vi "DBVI.vi"(8 "error in (no error)":errorcluster, 10 "ControlQueue":refnum<queue>, 11 "DB in":refnum<class "DB.lvclass">) -> (0 "error out":errorcluster)   [LabVIEW 2015, in "DB.lvclass"]
uses:
  DB.lvclass
  controls/Add.ctl
  controls/Del.ctl
  controls/Update.ctl
  controls/Fix.ctl
  dependecies/ControlsVIs/Clusters-def/Message types.ctl
  Def_DB_FP_ref_commands.ctl
  Def_fix_sql_param.ctl
  GeneralFunctionality/GeneralFunctionality.lvclass/GeneralFunctionality.ctl
  DB.lvclass/DB.ctl
  Message/Message.lvclass/Message.ctl
  dependecies/ControlsVIs/Clusters-def/Standard Command.ctl
  GeneralFunctionality/GeneralFunctionality.lvclass
  Message/Message.lvclass
panel:
  in  "Fix Exp Date":T1
  out "Result Set":string[][](table) caption="Result Set (from first statement with results)"
  in  "SQL command":string
  in  "Fix Users":T1
  in  "Fix Samples":T1=TRUE
  in  "Fix Project":T1=TRUE
  in  "Project Users":string
  in  "Project Date":string caption="Date"
  in  "Project Description":string caption="Description"
  in  "Projects":i16(ring) items=["GNP", "ND"]
  in  "Update project":T2
  in  "Del project":T3
  in  "Add Project":T4
  in  "Project Name":string caption="Name"
  in  "User Date":string caption="Date"
  in  "User  Description":string caption="Description"
  in  "Users":i16(ring) items=["Sergey", "Slava", "Mehran", "Raluca", "Pierre", "Jean-Philippe", "Audrey", "Furong", "Jean-Louis", "Isabelle", "Kash"]
  in  "Update User":T2
  in  "Del User":T3
  in  "Add User":T4
  in  "User name":string caption="Name"
  in  "Exp Date":string caption="Date"
  in  "Exp  Description":string caption="Description"
  in  "Experiments":i16(ring) items=["1-GNP-1_1mM"]
  in  "Update Exp":T2
  in  "Del Exp":T3
  in  "Add Exp":T4
  in  "Exp name":string caption="Name"
  in  "Sample Date":string caption="Date"
  in  "Sample Description":string caption="Description"
  in  "Samples":i16(ring) items=["GNP", "GNP-2mM"]
  in  "Update Sample":T2
  in  "Del Sample":T3
  in  "Add Sample":T4
  in  "Sample Name":string caption="Name"
  out "Received command":string
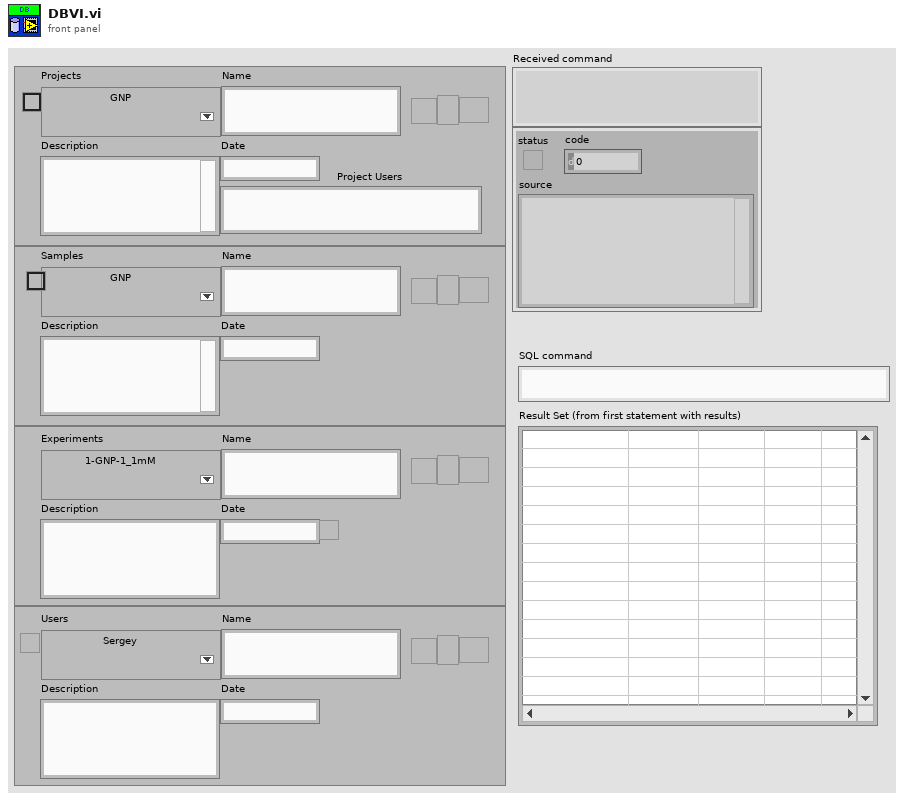
[diagram p1: front panel]
types:
  T1 = typedef "Fix.ctl" = bool
  T2 = typedef "Update.ctl" = bool
  T3 = typedef "Del.ctl" = bool
  T4 = typedef "Add.ctl" = bool
  T5 = typedef "DB.lvclass/Def_fix_sql_param.ctl" = cluster{"Fix Project":bool, "Fix Sample":bool, "Fix Exp Date":bool, "Fix User":bool}
  T6 = typedef "DB.lvclass/Def_DB_FP_ref_commands.ctl" = cluster{"Project Name":refnum<vi>, "Projects":refnum<vi>, "Project Description":refnum<vi>, "Project Date":refnum<vi>, "Project Users":refnum<vi>, "Samples":refnum<vi>, "Sample Name":refnum<vi>, "Sample Description":refnum<vi>, "Sample Date":refnum<vi>, "Experiments":refnum<vi>, "Exp Name":refnum<vi>, "Exp Description":refnum<vi>, "Exp Date":refnum<vi>, "Users":refnum<vi>, "User Name":refnum<vi>, "User Description":refnum<vi>, "User Date":refnum<vi>}
  T7 = typedef "Message types.ctl" = string
  T8 = typedef "Standard Command.ctl" = cluster{"command":string, "data":variant}
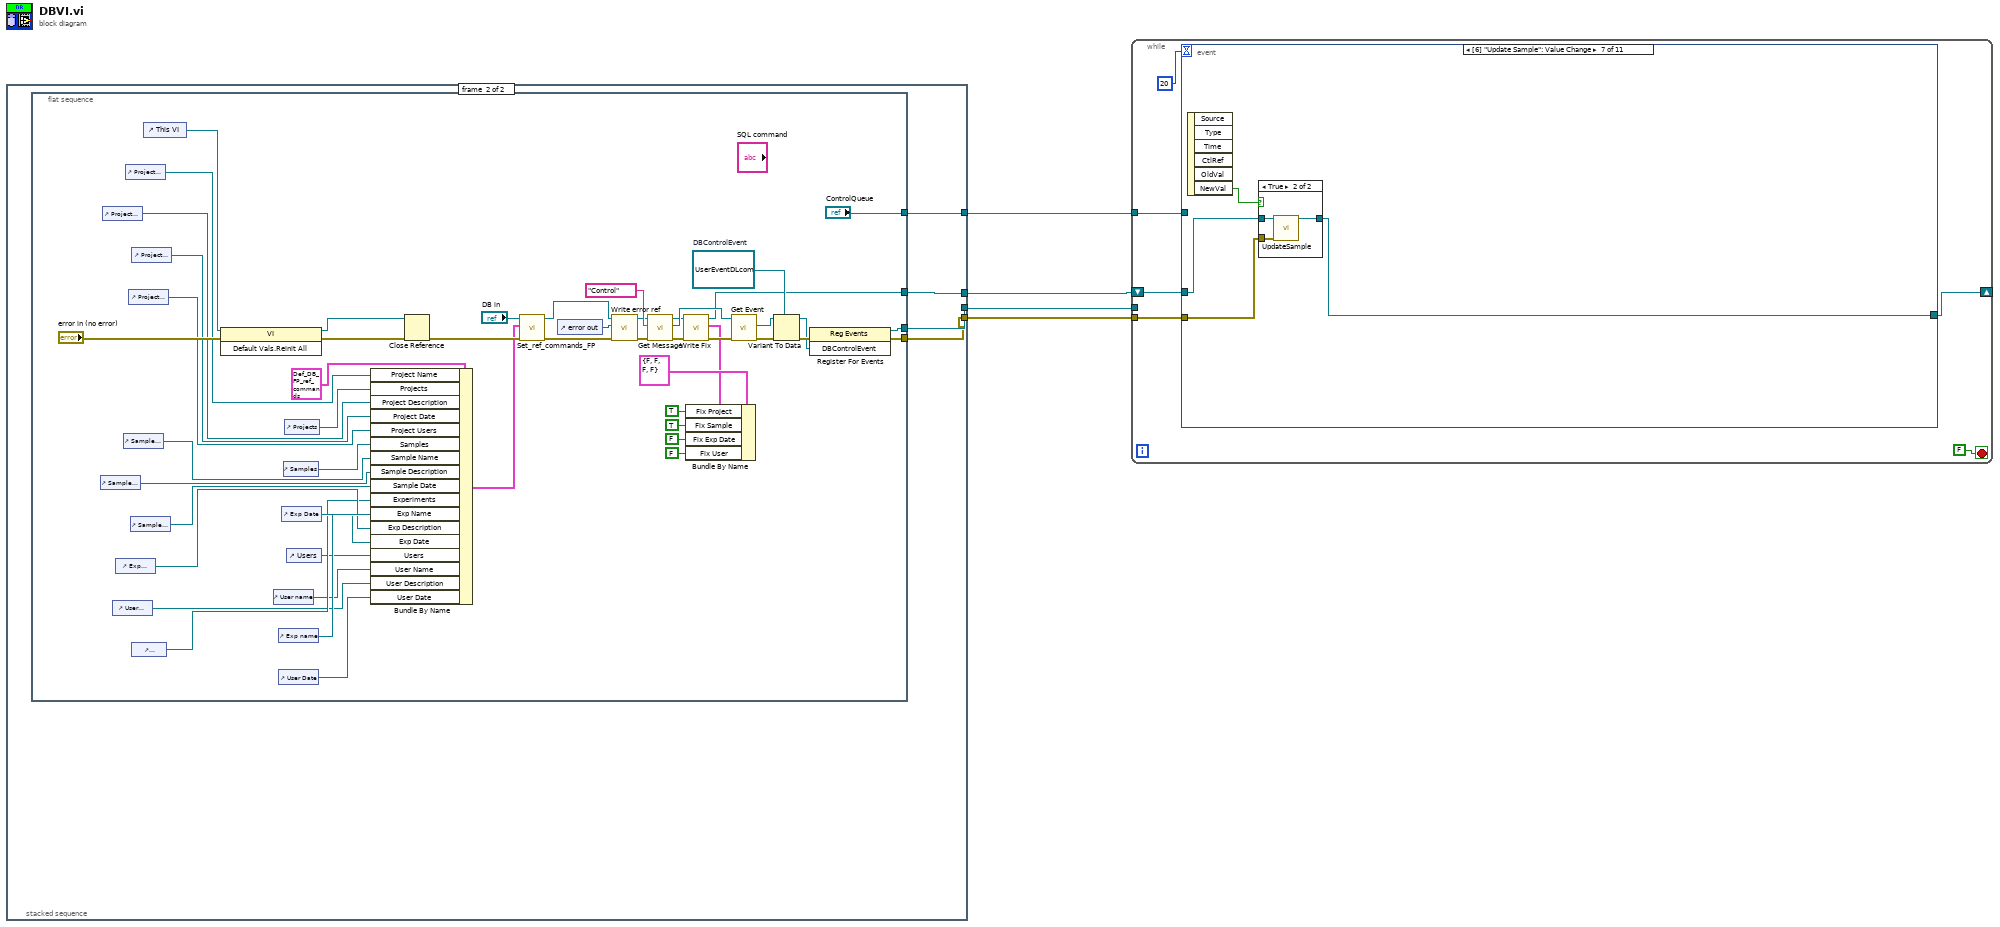
[diagram p0: block diagram]
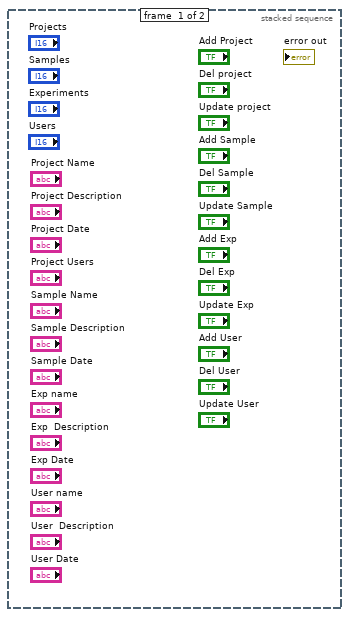
[diagram p2: hidden frame]
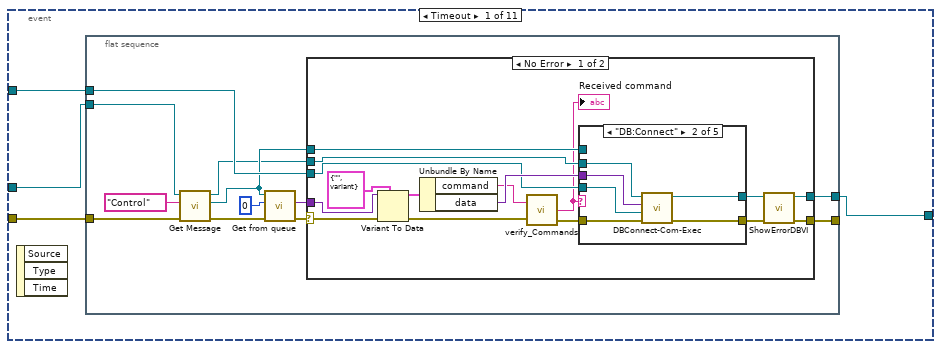
[diagram p3: hidden frame]
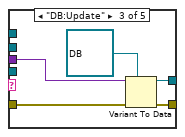
[diagram p5: hidden frame]
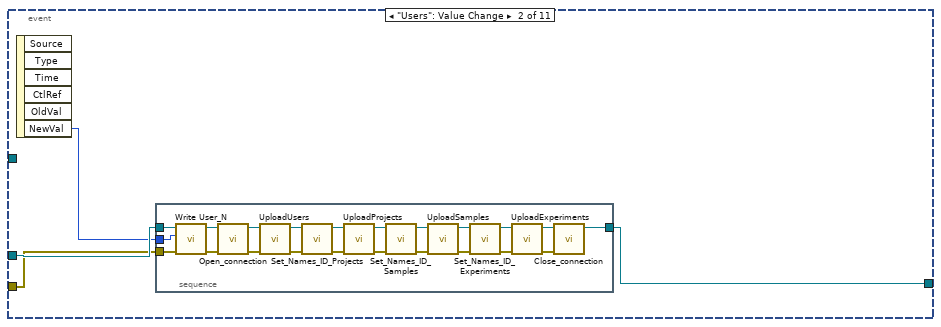
[diagram p9: hidden frame]
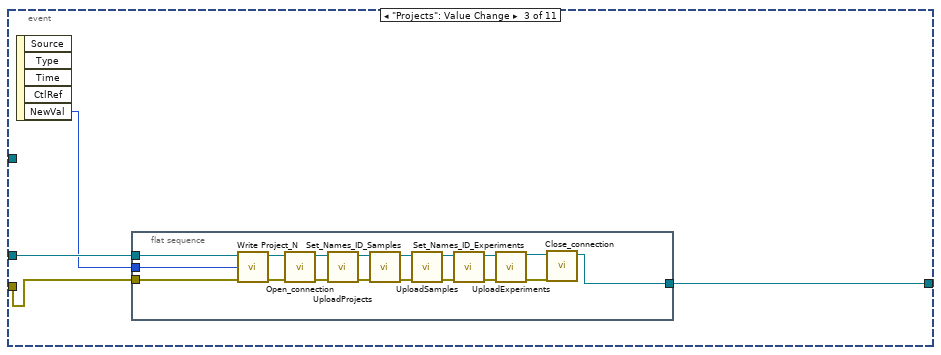
[diagram p10: hidden frame]
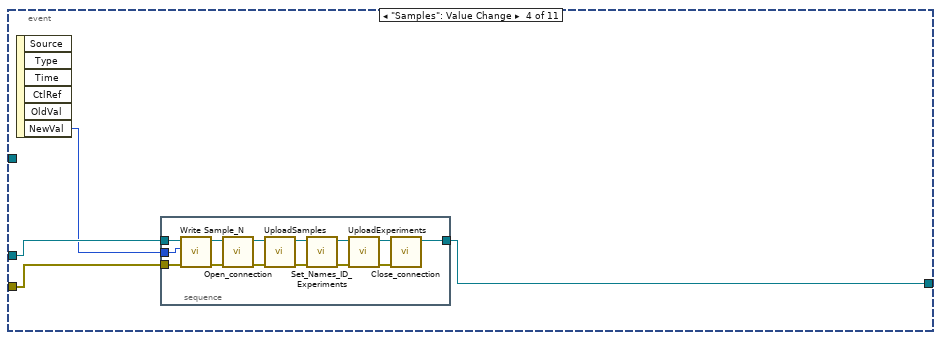
[diagram p11: hidden frame]
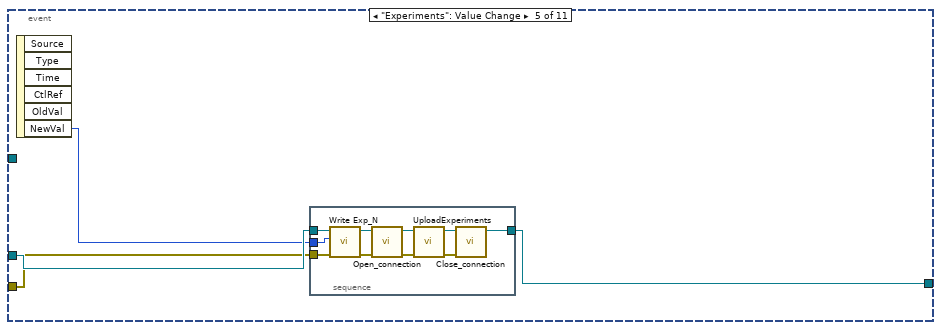
[diagram p12: hidden frame]
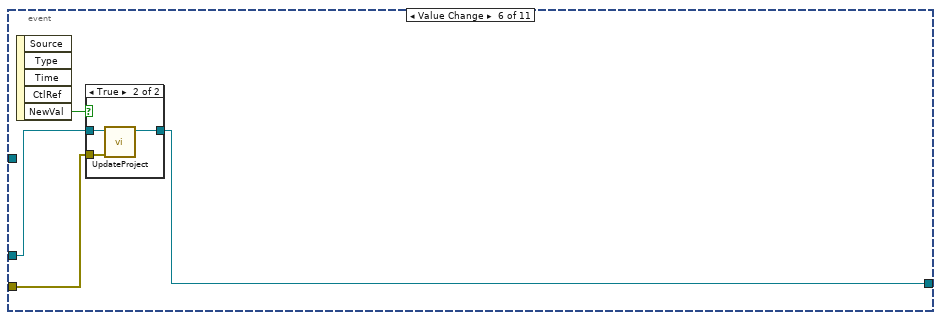
[diagram p13: hidden frame]
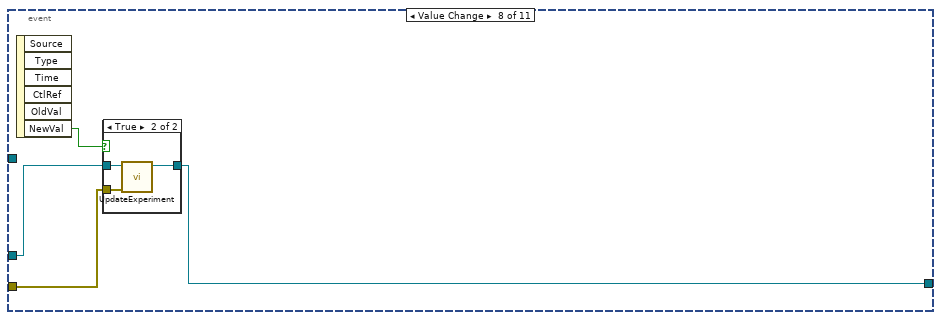
[diagram p16: hidden frame]
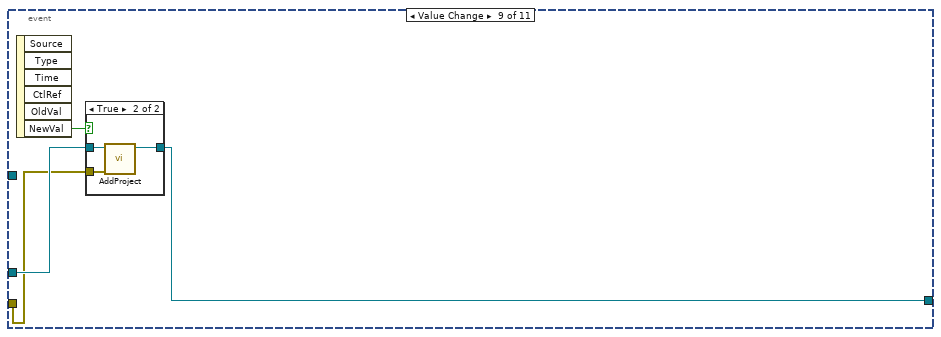
[diagram p18: hidden frame]
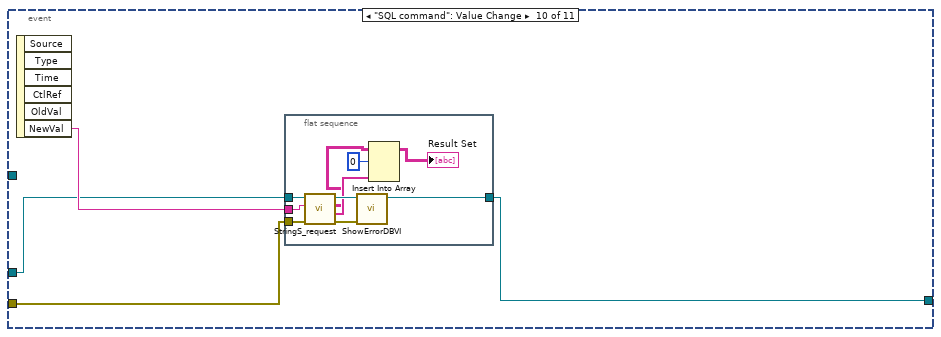
[diagram p20: hidden frame]
diagram:
  n1 = stacked-sequence {
    tunnel: [_ w5] -> w4
    tunnel: [_ w8] -> w1
    tunnel: [_ w6] -> w2
    tunnel: [_ w7] -> w3
    frame #0 {
    }
    frame #1 {
      n2 = flat-sequence {
        tunnel: [w17] -> w8
        tunnel: [w51] -> w7
        tunnel: [w50] -> w6
        tunnel: ["ControlQueue"] -> w5
        frame #0 {
          w49 = refnum<user-event> refnum  # DBControlEvent
          n3 = control-ref of="Sample Description"() -> (w29:refnum<vi>)
          n4 = control-ref of="Project Description"() -> (w33:refnum<vi>)
          n5 = control-ref of="User  Description"() -> (w21:refnum<vi>)
          n6 = control-ref of="Exp  Description"() -> (w26:refnum<vi>)
          n7 = control-ref of="Sample Name"() -> (w30:refnum<vi>)
          n8 = control-ref of="Project Name"() -> (w40:refnum<vi>)
          n9 = control-ref of="Project Users"() -> (w23:refnum<vi>)
          n10 = control-ref of="Sample Date"() -> (w28:refnum<vi>)
          n11 = control-ref of="Project Date"() -> (w32:refnum<vi>)
          n12 = control-ref of="Experiments"() -> (w24:refnum<vi>)
          n13 = control-ref of="This VI"() -> (w56:refnum<vi>)
          n14 = invoke class="VI" method="Default Vals.Reinit All"(reference=w56, error in="error in (no error)") -> (reference out=w57:refnum<vi>, error out=w58:errorcluster)  [unwired: 1 in, 1 out]
          n15 = control-ref of="User name"() -> (w20:refnum<vi>)
          n16 = control-ref of="Exp name"() -> (w27:refnum<vi>)
          n17 = control-ref of="User Date"() -> (w22:refnum<vi>)
          n18 = control-ref of="Exp Date"() -> (w25:refnum<vi>)
          n19 = control-ref of="Samples"() -> (w31:refnum<vi>)
          n20 = control-ref of="Projects"() -> (w39:refnum<vi>)
          n21 = control-ref of="Users"() -> (w19:refnum<vi>)
          n22 = Bundle By Name(cluster=T6 {"Project Name"=refnum, "Projects"=refnum, "Project Description"=refnum, "Project Date"=refnum, "Project Users"=refnum, "Samples"=refnum, "Sample Name"=refnum, "Sample Description"=refnum, "Sample Date"=refnum, "Experiments"=refnum, "Exp Name"=refnum, "Exp Description"=refnum, "Exp Date"=refnum, "Users"=refnum, "User Name"=refnum, "User Description"=refnum, "User Date"=refnum}, "Project Name"=w40, "Projects"=w39, "Project Description"=w33, "Project Date"=w32, "Project Users"=w23, "Samples"=w31, "Sample Name"=w30, "Sample Description"=w29, "Sample Date"=w28, "Experiments"=w24, "Exp Name"=w27, "Exp Description"=w26, "Exp Date"=w25, "Users"=w19, "User Name"=w20, "User Description"=w21, "User Date"=w22) -> (w34:T6)
          n23 = Close Reference(reference=w57, error in (no error)=w58) -> (error out=w35:errorcluster)
          n24 = call "Set_ref_commands_FP.vi"("error in (no error)"=w35, "controls_refs"=w34, "DB in"="DB in") -> ("error out"=w38:errorcluster, "DB out"=w37:refnum<class "DB.lvclass">)  [unwired: 7 in]
          n25 = control-ref of="error out"() -> (w43:refnum<vi>)
          n26 = call "Write error ref.vi"("error in (no error)"=w38, "error"=w43, "GeneralFunctionality in"=w37) -> ("error out"=w53:errorcluster, "GeneralFunctionality out"=w54:refnum<class "DB.lvclass">)  [unwired: 7 in]
          n27 = call "Get Message.vi"("error in (no error)"=w53, "Message type"=T7 "Control", "GeneralFunctionality en entrée"=w54) -> ("error out"=w16:errorcluster, "Message.lvclass"=w52:refnum<class "Message.lvclass">, "GeneralFunctionality en sortie"=w18:refnum<class "DB.lvclass">)  [unwired: 6 in]
          n28 = Bundle By Name(cluster=T5 {"Fix Project"=FALSE, "Fix Sample"=FALSE, "Fix Exp Date"=FALSE, "Fix User"=FALSE}, "Fix Project"=TRUE, "Fix Sample"=TRUE, "Fix Exp Date"=FALSE, "Fix User"=FALSE) -> (w9:T5)
          n29 = call "Write Fix.vi"("error in (no error)"=w16, "Fix"=w9, "DB in"=w18) -> ("error out"=w15:errorcluster, "DB out"=w17:refnum<class "DB.lvclass">)  [unwired: 7 in]
          n30 = call "Get Event.vi"("error in (no error)"=w15, "Message en entrée"=w52) -> ("error out"=w48:errorcluster, "UserEventCommand"=w46:refnum<user-event>)  [unwired: 7 in, 1 out]
          n31 = Variant To Data(error in=w48, type=w49, Variant=w46) -> (data=w45:refnum<user-event>, error out=w47:errorcluster)
          n32 = register-events(error in=w47, w45) -> (reference out=w51:refnum<event-registration>, error out=w50:errorcluster)  [unwired: 1 in]
        }
      }
    }
  }
  n33 = while {
    tunnel: w4 -> [w64]
    tunnel: w3 -> [_]
    tunnel: w2 -> [w63]
    shift-right: [w59] -> _
    shift-left: w1 -> [w62]
    stop <- FALSE stop-if-true
    n34 = event shown="[6] \"Update Sample\": Value Change" {
      selector: _ -> [_ _ _ _ _ _ _ _ _ _ _]
      dyn-events: _ -> [_ _ _ _ _ _ _ _ _ _ _]
      timeout: 20 -> [_ _ _ _ _ _ _ _ _ _ _]
      tunnel: w64 -> [w68 _ _ _ _ _ _ _ _ _ _]
      tunnel: w63 -> [w67 w118 w144 w167 w183 w199 w205 w213 w222 w230 w243]
      tunnel: w62 -> [w66 w119 w145 w166 w185 w198 w206 w214 w223 w229 w244]
      tunnel: [w65 w116 w142 w164 w182 w196 w204 w212 w220 w228 w242] -> w59
      event Timeout {
        n35 = event-data() -> ()  [unwired: 1 in, 3 out]
        n36 = flat-sequence {
          tunnel: [w77] -> w65
          tunnel: [w76] -> _
          tunnel: w68 -> [w75]
          tunnel: w66 -> [w71]
          tunnel: w67 -> [w70]
          frame #0 {
            n37 = call "Get Message.vi"("error in (no error)"=w70, "Message type"=T7 "Control", "GeneralFunctionality en entrée"=w71) -> ("error out"=w74:errorcluster, "Message.lvclass"=w73:refnum<class "Message.lvclass">, "GeneralFunctionality en sortie"=w69:refnum<class "DB.lvclass">)  [unwired: 6 in]
            n38 = call "Get from queue.vi"("error in (no error)"=w74, "timeout in ms (-1)"=0, "Message in"=w73) -> ("error out"=w78:errorcluster, "Data"=w79:variant)  [unwired: 6 in, 1 out]
            n39 = case shown="No Error" w78 {
              selector: w78 -> [w96 w114]
              tunnel: w79 -> [w90 _]
              tunnel: [w84 w114] -> w76
              tunnel: w69 -> [w92 w115]
              tunnel: [w83 w115] -> w77
              tunnel: w75 -> [w91 _]
              tunnel: w73 -> [w89 _]
              frame No Error {
                n40 = Variant To Data(error in=w96, type=T8 {"command"="", "data"=variant} ("input cluster"), Variant=w90) -> (data=w94:T8, error out=w87:errorcluster)
                n41 = Unbundle By Name(w94) -> ("command"=w88:string, "data"=w93:variant)
                n42 = call "verify_Commands.vi"("Command"=w88, "error in"=w87) -> ("Command out"=w85:string, "error out"=w86:errorcluster)  [unwired: 1 out]
                "Received command" <- w85
                n43 = case shown="\"DB:Connect\"" w85 {
                  tunnel: [w98 w102 w106 w111 w113] -> w81
                  tunnel: [w97 w103 w107 w110 w112] -> w82
                  tunnel: w93 -> [_ w100 w109 _ _]
                  tunnel: w86 -> [w97 w104 w108 w110 w112]
                  tunnel: w92 -> [w98 w99 _ w111 w113]
                  tunnel: w91 -> [_ w101 _ _ _]
                  tunnel: w89 -> [_ _ _ _ _]
                  frame "Error", Default {
                  }
                  frame "DB:Connect" {
                    n44 = call "DBConnect-Com-Exec.vi"("error in (no error)"=w104, "ControlQueue"=w101, "data"=w100, "DB in"=w99) -> ("error out"=w103:errorcluster, "DB out"=w102:refnum<class "DB.lvclass">)  [unwired: 6 in]
                  }
                  frame "DB:Update" {
                    n45 = Variant To Data(error in=w108, type=refnum<class "DB.lvclass"> refnum ("DB.lvclass"), Variant=w109) -> (data=w106:refnum<class "DB.lvclass">, error out=w107:errorcluster)
                  }
                  frame "DB:Status" {
                  }
                  frame "DB:SQL" {
                  }
                }
                n46 = call "ShowErrorDBVI.vi"("error in (no error)"=w82, "DB in"=w81) -> ("error out"=w84:errorcluster, "DB out"=w83:refnum<class "DB.lvclass">)  [unwired: 8 in]
              }
              frame Error {
              }
            }
          }
        }
      }
      event "Users": Value Change {
        n47 = event-data() -> ("NewVal"=w117:i16)  [unwired: 1 in, 5 out]
        n48 = stacked-sequence {
          tunnel: w118 -> [w141]
          tunnel: w119 -> [w140]
          tunnel: w117 -> [w139]
          tunnel: [w126] -> w116
          frame #0 {
            n49 = call "Write User_N.vi"("error in (no error)"=w141, "Exp_N"=w139, "DB in"=w140) -> ("error out"=w124:errorcluster, "DB out"=w121:refnum<class "DB.lvclass">)  [unwired: 7 in]
            n50 = call-dynamic "Open_connection.vi"("error in (no error)"=w124, "DB in"=w121) -> ("error out"=w123:errorcluster, "DB out"=w122:refnum<class "DB.lvclass">)  [unwired: 8 in]
            n51 = call "UploadUsers.vi"("error in (no error)"=w123, "DB in"=w122) -> ("error out"=w128:errorcluster, "DB out"=w129:refnum<class "DB.lvclass">)  [unwired: 8 in]
            n52 = call "Set_Names_ID_Projects.vi"("error in (no error)"=w128, "DB in"=w129) -> ("error out"=w120:errorcluster, "DB out"=w130:refnum<class "DB.lvclass">)  [unwired: 8 in]
            n53 = call "UploadProjects.vi"("error in (no error)"=w120, "DB in"=w130) -> ("error out"=w131:errorcluster, "DB out"=w132:refnum<class "DB.lvclass">)  [unwired: 8 in]
            n54 = call "Set_Names_ID_Samples.vi"("error in (no error)"=w131, "DB in"=w132) -> ("error out"=w133:errorcluster, "DB out"=w134:refnum<class "DB.lvclass">)  [unwired: 8 in]
            n55 = call "UploadSamples.vi"("error in (no error)"=w133, "DB in"=w134) -> ("error out"=w135:errorcluster, "DB out"=w136:refnum<class "DB.lvclass">)  [unwired: 8 in]
            n56 = call "Set_Names_ID_Experiments.vi"("error in (no error)"=w135, "DB in"=w136) -> ("error out"=w138:errorcluster, "DB out"=w137:refnum<class "DB.lvclass">)  [unwired: 8 in]
            n57 = call "UploadExperiments.vi"("error in (no error)"=w138, "DB in"=w137) -> ("error out"=w127:errorcluster, "DB out"=w125:refnum<class "DB.lvclass">)  [unwired: 8 in]
            n58 = call-dynamic "Close_connection.vi"("error in (no error)"=w127, "DB in"=w125) -> ("DB out"=w126:refnum<class "DB.lvclass">)  [unwired: 8 in, 1 out]
          }
        }
      }
      event "Projects": Value Change {
        n59 = event-data() -> ("NewVal"=w143:i16)  [unwired: 1 in, 4 out]
        n60 = flat-sequence {
          tunnel: w145 -> [w163]
          tunnel: w144 -> [w162]
          tunnel: w143 -> [w161]
          tunnel: [w146] -> w142
          frame #0 {
            n61 = call "Write Project_N.vi"("error in (no error)"=w162, "Project_id"=w161, "DB in"=w163) -> ("error out"=w152:errorcluster, "DB out"=w151:refnum<class "DB.lvclass">)  [unwired: 7 in]
            n62 = call-dynamic "Open_connection.vi"("error in (no error)"=w152, "DB in"=w151) -> ("error out"=w149:errorcluster, "DB out"=w150:refnum<class "DB.lvclass">)  [unwired: 8 in]
            n63 = call "UploadProjects.vi"("error in (no error)"=w149, "DB in"=w150) -> ("error out"=w160:errorcluster, "DB out"=w159:refnum<class "DB.lvclass">)  [unwired: 8 in]
            n64 = call "Set_Names_ID_Samples.vi"("error in (no error)"=w160, "DB in"=w159) -> ("error out"=w158:errorcluster, "DB out"=w157:refnum<class "DB.lvclass">)  [unwired: 8 in]
            n65 = call "UploadSamples.vi"("error in (no error)"=w158, "DB in"=w157) -> ("error out"=w156:errorcluster, "DB out"=w155:refnum<class "DB.lvclass">)  [unwired: 8 in]
            n66 = call "Set_Names_ID_Experiments.vi"("error in (no error)"=w156, "DB in"=w155) -> ("error out"=w153:errorcluster, "DB out"=w154:refnum<class "DB.lvclass">)  [unwired: 8 in]
            n67 = call "UploadExperiments.vi"("error in (no error)"=w153, "DB in"=w154) -> ("error out"=w148:errorcluster, "DB out"=w147:refnum<class "DB.lvclass">)  [unwired: 8 in]
            n68 = call-dynamic "Close_connection.vi"("error in (no error)"=w148, "DB in"=w147) -> ("DB out"=w146:refnum<class "DB.lvclass">)  [unwired: 8 in, 1 out]
          }
        }
      }
      event "Samples": Value Change {
        n69 = event-data() -> ("NewVal"=w165:i16)  [unwired: 1 in, 5 out]
        n70 = stacked-sequence {
          tunnel: w167 -> [w181]
          tunnel: w166 -> [w180]
          tunnel: [w173] -> w164
          tunnel: w165 -> [w179]
          frame #0 {
            n71 = call "Write Sample_N.vi"("error in (no error)"=w181, "Sample_N"=w179, "DB in"=w180) -> ("error out"=w168:errorcluster, "DB out"=w171:refnum<class "DB.lvclass">)  [unwired: 7 in]
            n72 = call-dynamic "Open_connection.vi"("error in (no error)"=w168, "DB in"=w171) -> ("error out"=w169:errorcluster, "DB out"=w170:refnum<class "DB.lvclass">)  [unwired: 8 in]
            n73 = call "UploadSamples.vi"("error in (no error)"=w169, "DB in"=w170) -> ("error out"=w175:errorcluster, "DB out"=w177:refnum<class "DB.lvclass">)  [unwired: 8 in]
            n74 = call "Set_Names_ID_Experiments.vi"("error in (no error)"=w175, "DB in"=w177) -> ("error out"=w178:errorcluster, "DB out"=w176:refnum<class "DB.lvclass">)  [unwired: 8 in]
            n75 = call "UploadExperiments.vi"("error in (no error)"=w178, "DB in"=w176) -> ("error out"=w172:errorcluster, "DB out"=w174:refnum<class "DB.lvclass">)  [unwired: 8 in]
            n76 = call-dynamic "Close_connection.vi"("error in (no error)"=w172, "DB in"=w174) -> ("DB out"=w173:refnum<class "DB.lvclass">)  [unwired: 8 in, 1 out]
          }
        }
      }
      event "Experiments": Value Change {
        n77 = event-data() -> ("NewVal"=w184:i16)  [unwired: 1 in, 5 out]
        n78 = stacked-sequence {
          tunnel: w183 -> [w195]
          tunnel: w185 -> [w194]
          tunnel: [w191] -> w182
          tunnel: w184 -> [w193]
          frame #0 {
            n79 = call "Write Exp_N.vi"("error in (no error)"=w195, "Exp_N"=w193, "DB in"=w194) -> ("error out"=w186:errorcluster, "DB out"=w189:refnum<class "DB.lvclass">)  [unwired: 7 in]
            n80 = call-dynamic "Open_connection.vi"("error in (no error)"=w186, "DB in"=w189) -> ("error out"=w187:errorcluster, "DB out"=w188:refnum<class "DB.lvclass">)  [unwired: 8 in]
            n81 = call "UploadExperiments.vi"("error in (no error)"=w187, "DB in"=w188) -> ("error out"=w190:errorcluster, "DB out"=w192:refnum<class "DB.lvclass">)  [unwired: 8 in]
            n82 = call-dynamic "Close_connection.vi"("error in (no error)"=w190, "DB in"=w192) -> ("DB out"=w191:refnum<class "DB.lvclass">)  [unwired: 8 in, 1 out]
          }
        }
      }
      event Value Change {
        n83 = event-data() -> ("NewVal"=w197:T2)  [unwired: 1 in, 4 out]
        n84 = case shown="True" w197 {
          tunnel: w199 -> [_ w203]
          tunnel: w198 -> [w200 w202]
          tunnel: [w200 w201] -> w196
          frame False {
          }
          frame True {
            n85 = call-dynamic "UpdateProject.vi"("error in (no error)"=w203, "DB in"=w202) -> ("DB out"=w201:refnum<class "DB.lvclass">)  [unwired: 8 in, 1 out]
          }
        }
      }
      event Value Change {
        n86 = event-data() -> ("NewVal"=w207:T2)  [unwired: 1 in, 5 out]
        n87 = case shown="True" w207 {
          tunnel: w205 -> [_ w211]
          tunnel: w206 -> [w208 w210]
          tunnel: [w208 w209] -> w204
          frame False {
          }
          frame True {
            n88 = call-dynamic "UpdateSample.vi"("error in (no error)"=w211, "DB in"=w210) -> ("DB out"=w209:refnum<class "DB.lvclass">)  [unwired: 8 in, 1 out]
          }
        }
      }
      event Value Change {
        n89 = event-data() -> ("NewVal"=w215:T2)  [unwired: 1 in, 5 out]
        n90 = case shown="True" w215 {
          tunnel: w213 -> [_ w219]
          tunnel: w214 -> [w216 w218]
          tunnel: [w216 w217] -> w212
          frame False {
          }
          frame True {
            n91 = call-dynamic "UpdateExperiment.vi"("error in (no error)"=w219, "DB in"=w218) -> ("DB out"=w217:refnum<class "DB.lvclass">)  [unwired: 8 in, 1 out]
          }
        }
      }
      event Value Change {
        n92 = event-data() -> ("NewVal"=w221:T4)  [unwired: 1 in, 5 out]
        n93 = case shown="True" w221 {
          tunnel: w223 -> [w224 w227]
          tunnel: [w224 w226] -> w220
          tunnel: w222 -> [_ w225]
          frame False {
          }
          frame True {
            n94 = call "AddProject.vi"("error in (no error)"=w225, "DB in"=w227) -> ("DB out"=w226:refnum<class "DB.lvclass">)  [unwired: 8 in, 1 out]
          }
        }
      }
      event "SQL command": Value Change {
        n95 = event-data() -> ("NewVal"=w231:string)  [unwired: 1 in, 5 out]
        n96 = flat-sequence {
          tunnel: w231 -> [w241]
          tunnel: w230 -> [w240]
          tunnel: w229 -> [w239]
          tunnel: [w237] -> w228
          frame #0 {
            n97 = call-dynamic "StringS_request.vi"("error in (no error)"=w240, "SQL request"=w241, "DB in"=w239) -> ("error out"=w238:errorcluster, "Column Names"=w235:string[], "Result Set"=w233:string[][], "DB out"=w236:refnum<class "DB.lvclass">)  [unwired: 5 in]
            n98 = call "ShowErrorDBVI.vi"("error in (no error)"=w238, "DB in"=w236) -> ("DB out"=w237:refnum<class "DB.lvclass">)  [unwired: 8 in, 1 out]
            n99 = Insert Into Array(array=w233, index (row)=0 ("index"), new element=w235) -> (→"Result Set":string[][])  [unwired: 1 in]
          }
        }
      }
      event Value Change {
        n100 = event-data() -> ()  [unwired: 1 in, 6 out]
        n101 = flat-sequence {
          tunnel: w244 -> [w255]
          tunnel: w243 -> [w254]
          tunnel: [w245] -> w242
          frame #0 {
            n102 = Bundle By Name(cluster=T5 {"Fix Project"=FALSE, "Fix Sample"=FALSE, "Fix Exp Date"=FALSE, "Fix User"=FALSE}, "Fix Project"="Fix Project", "Fix Sample"="Fix Samples", "Fix Exp Date"="Fix Exp Date", "Fix User"="Fix Users") -> (w248:T5)
            n103 = call "Write Fix.vi"("error in (no error)"=w254, "Fix"=w248, "DB in"=w255) -> ("error out"=w247:errorcluster, "DB out"=w246:refnum<class "DB.lvclass">)  [unwired: 7 in]
            n104 = flat-sequence {
              tunnel: w247 -> [w259]
              tunnel: [w260] -> w245
              tunnel: w246 -> [w256]
              frame #0 {
                n105 = call-dynamic "Open_connection.vi"("error in (no error)"=w259, "DB in"=w256) -> ("error out"=w258:errorcluster, "DB out"=w257:refnum<class "DB.lvclass">)  [unwired: 8 in]
                n106 = call "Set_Names_ID_Projects.vi"("error in (no error)"=w258, "DB in"=w257) -> ("error out"=w264:errorcluster, "DB out"=w263:refnum<class "DB.lvclass">)  [unwired: 8 in]
                n107 = call "UploadProjects.vi"("error in (no error)"=w264, "DB in"=w263) -> ("error out"=w272:errorcluster, "DB out"=w271:refnum<class "DB.lvclass">)  [unwired: 8 in]
                n108 = call "Set_Names_ID_Samples.vi"("error in (no error)"=w272, "DB in"=w271) -> ("error out"=w270:errorcluster, "DB out"=w269:refnum<class "DB.lvclass">)  [unwired: 8 in]
                n109 = call "UploadSamples.vi"("error in (no error)"=w270, "DB in"=w269) -> ("error out"=w268:errorcluster, "DB out"=w267:refnum<class "DB.lvclass">)  [unwired: 8 in]
                n110 = call "Set_Names_ID_Experiments.vi"("error in (no error)"=w268, "DB in"=w267) -> ("error out"=w265:errorcluster, "DB out"=w266:refnum<class "DB.lvclass">)  [unwired: 8 in]
                n111 = call "UploadExperiments.vi"("error in (no error)"=w265, "DB in"=w266) -> ("error out"=w262:errorcluster, "DB out"=w261:refnum<class "DB.lvclass">)  [unwired: 8 in]
                n112 = call-dynamic "Close_connection.vi"("error in (no error)"=w262, "DB in"=w261) -> ("DB out"=w260:refnum<class "DB.lvclass">)  [unwired: 8 in, 1 out]
              }
            }
          }
        }
      }
    }
  }
